vi "Interpolate 2D Scattered (1D).vi"(6 "Yi":dbl[](array[numeric]), 7 "method":i32(ring)=1 items=["nearest", "linear", "cubic", "biharmonic spline "], 8 "Xi":dbl[](array[numeric]), 9 "Y":dbl[](array[numeric]), 10 "X":dbl[](array[numeric]), 11 "Z":dbl[](array[numeric])) -> (0 "error":i32, 3 "Zi":dbl[](array[numeric]))   [LabVIEW 2020, in "NI_AAL_Interpolation.lvlib"]
doc: "Performs two-dimensional interpolation on scattered points."
uses:
  <vilib>/gmath/NI_AAL_Interpolation.lvlib
panel:
  # "Interpolate 2D Scattered (1D)"
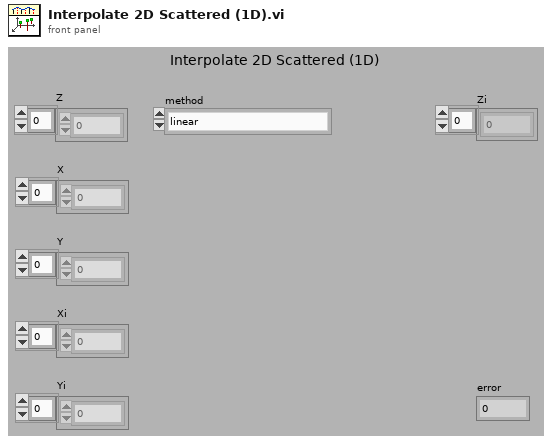
[diagram p1: front panel]
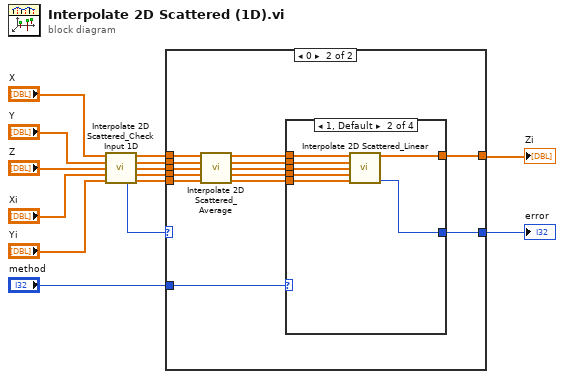
[diagram p0: block diagram]
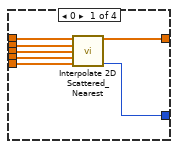
[diagram p3: hidden frame]
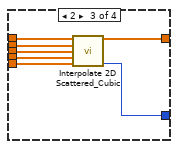
[diagram p4: hidden frame]
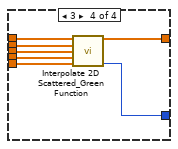
[diagram p5: hidden frame]
diagram:
  n1 = call <vilib>:"Interpolate 2D Scattered_Check Input 1D.vi"("X In"="X", "Y In"="Y", "Z In"="Z", "Xi In"="Xi", "Yi In"="Yi") -> ("X Out"=w7:dbl[], "Y Out"=w6:dbl[], "Z Out"=w5:dbl[], "Xi Out"=w4:dbl[], "error"=w2:i32, "Yi Out"=w3:dbl[])  [unwired: 5 out]
  n2 = case shown="0" w2 {
    selector: w2 -> [w15 _]
    tunnel: "method" -> [_ w28]
    tunnel: [_ w24] -> w13
    tunnel: w7 -> [_ w21]
    tunnel: w6 -> [_ w20]
    tunnel: w5 -> [_ w19]
    tunnel: w4 -> [_ w18]
    tunnel: w3 -> [_ w17]
    tunnel: [w15 w16] -> w1
    frame -1, Default {
    }
    frame 0 {
      n3 = call <vilib>:"Interpolate 2D Scattered_Average.vi"("X In"=w21, "Y In"=w20, "Z In"=w19, "Xi In"=w18, "Yi In"=w17) -> ("X Out"=w27:dbl[], "Y Out"=w26:dbl[], "Z Out"=w25:dbl[], "Xi Out"=w23:dbl[], "Yi Out"=w22:dbl[])  [unwired: 6 out]
      n4 = case shown="1, Default" w28 {
        tunnel: w27 -> [w35 w42 w49 w56]
        tunnel: w26 -> [w34 w41 w48 w55]
        tunnel: w25 -> [w33 w40 w47 w54]
        tunnel: w23 -> [w32 w39 w46 w53]
        tunnel: w22 -> [w31 w38 w45 w52]
        tunnel: [w29 w36 w43 w50] -> w24
        tunnel: [w30 w37 w44 w51] -> w16
        frame 0 {
          n5 = call <vilib>:"Interpolate 2D Scattered_Nearest.vi"("X"=w35, "Y"=w34, "Z"=w33, "Xi"=w32, "Yi"=w31) -> ("Zi"=w29:dbl[], "error"=w30:i32)  [unwired: 9 out]
        }
        frame 1, Default {
          n6 = call <vilib>:"Interpolate 2D Scattered_Linear.vi"("X"=w42, "Y"=w41, "Z"=w40, "Xi"=w39, "Yi"=w38) -> ("Zi"=w36:dbl[], "error"=w37:i32)  [unwired: 9 out]
        }
        frame 2 {
          n7 = call <vilib>:"Interpolate 2D Scattered_Cubic.vi"("X"=w49, "Y"=w48, "Z"=w47, "Xi"=w46, "Yi"=w45) -> ("Zi"=w43:dbl[], "error"=w44:i32)  [unwired: 9 out]
        }
        frame 3 {
          n8 = call <vilib>:"Interpolate 2D Scattered_Green Function.vi"("X"=w56, "Y"=w55, "Z"=w54, "Xi"=w53, "Yi"=w52) -> ("Zi"=w50:dbl[], "error"=w51:i32)  [unwired: 9 out]
        }
      }
    }
  }
  "Zi" <- w13
  "error" <- w1
